vi "dataProcess_spectrZeroOut.vi"(0 "reference":refnum<class "OSA.lvclass">, 1 "spectrum":sgl[](array[numeric]) format="%.2f", 2 "idx start":u32, 3 "idx stop":u32, 4 "length":u32, 5 "error in (no error)":errorcluster) -> (14 "duplicate reference":refnum<class "OSA.lvclass">, 19 "error out":errorcluster)   [LabVIEW 2010, in "OSA.lvclass"]
doc: "This zeros-out a spectrum between the two given indices On return will spectrum be equal to zero at and between the two indices, (idx_start, idx_stop)."
uses:
  OSA.lvclass
  typeDef/xVal_option.ctl
  OSA20X_misc.lvlib
  FTSLib.dll
panel:
  out "spectrum blanked":sgl[](array[numeric]) format="%.2f"
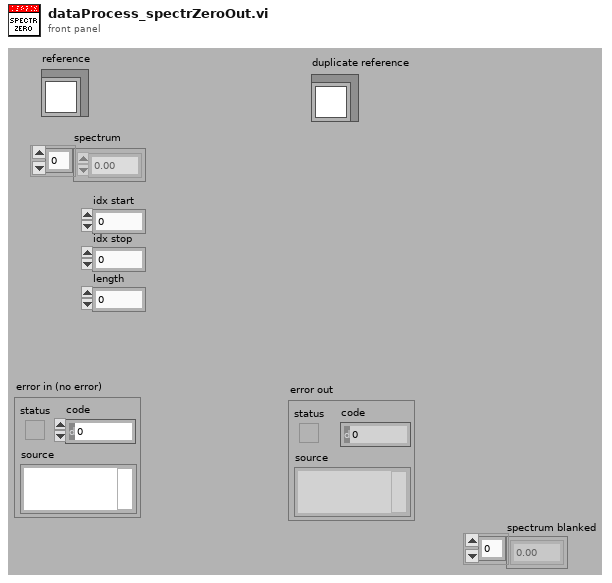
[diagram p1: front panel]
types:
  T1 = typedef "OSA.lvclass/xVal_option.ctl" = enum16{"MIN_MAX", "ARRAY"}
  T2 = cluster{"length":u32, "X min":sgl, "X max":sgl, "X_VAL_OPTIONS":T1}
  T3 = enum16{"get", "init", "set interferogram", "set spectrum", "cleanUp"}
  T4 = typedef "OSA.lvclass/spectrum_properties.ctl" = cluster{"length":u32, "X min":sgl, "X max":sgl, "X_VAL_OPTIONS":T1}
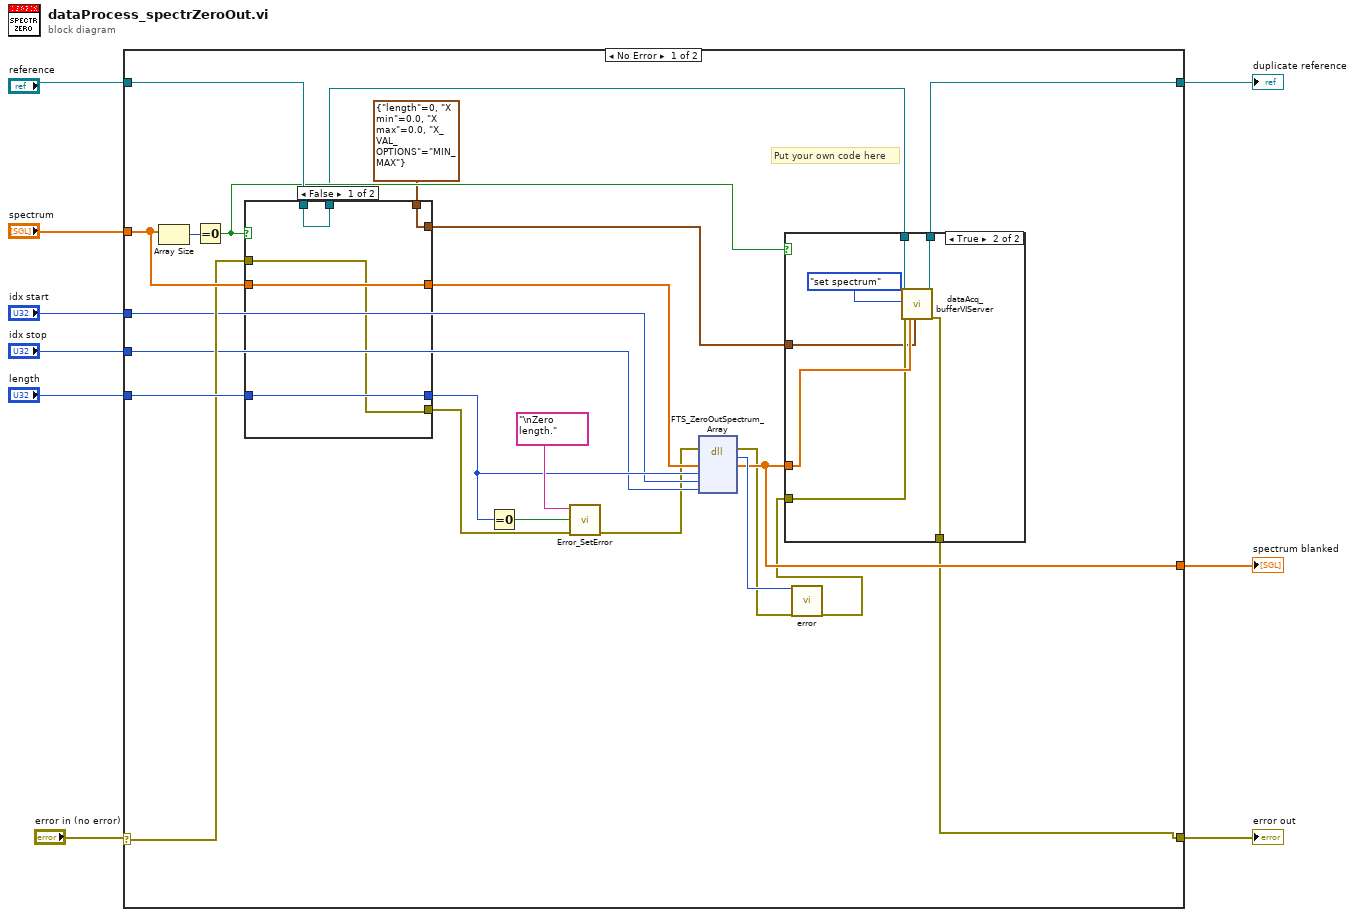
[diagram p0: block diagram]
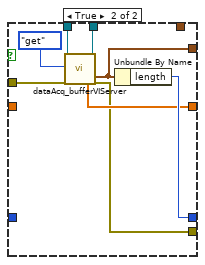
[diagram p3: hidden frame]
diagram:
  n1 = case shown="No Error" "error in (no error)" {
    selector: "error in (no error)" -> [w25 w56]
    tunnel: [w13 w56] -> w9
    tunnel: "reference" -> [w24 w57]
    tunnel: [w17 w57] -> w6
    tunnel: "spectrum" -> [w30 w55]
    tunnel: "idx start" -> [w21 _]
    tunnel: "idx stop" -> [w20 _]
    tunnel: "length" -> [w29 _]
    tunnel: [w16 w55] -> w1
    frame No Error {
      # "Put your own code here"
      n2 = Array Size(array=w30) -> (size(s)=w31:i32)
      n3 = Equal To 0?(x=w31) -> (x = 0?=w19:bool)
      n4 = case shown="False" w19 {
        tunnel: w30 -> [w46 _]
        tunnel: w29 -> [w45 _]
        tunnel: [w46 w50] -> w28
        tunnel: w24 -> [w44 w53]
        tunnel: [w44 w52] -> w18
        tunnel: w25 -> [w43 w48]
        tunnel: [w43 w47] -> w26
        tunnel: [w45 w54] -> w22
        tunnel: [w42 w51] -> w15
        tunnel: T2 {"length"=0, "X min"=0.0, "X max"=0.0, "X_VAL_OPTIONS"=enum."MIN_MAX"} ("spectrum property") -> [w42 _]
        frame False {
        }
        frame True {
          n5 = call "dataAcq_bufferVIServer.vi"("reference"=w53, "action"=T3."get", "error in (no error)"=w48) -> ("spectrum Y"=w50:sgl[], "duplicate reference"=w52:refnum<class "OSA.lvclass">, "spectrum prop"=w51:T4, "error out"=w47:errorcluster)  [unwired: 9 in, 4 out]
          n6 = Unbundle By Name(w51) -> ("length"=w54:u32)
        }
      }
      n7 = Equal To 0?(x=w22) -> (x = 0?=w23:bool)
      n8 = call "Error_SetError.vi"("error in"=w26, "status (true)"=w23, "source(\"\")"="\nZero length." ("source(\"\")")) -> ("error out"=w12:errorcluster)  [unwired: 4 in]
      n9 = dll-call lib="FTSLib.dll" fn="FTS_ZeroOutSpectrum_Array"(error in=w12, "spectrum"=w28, "length"=w22, "startIdx"=w21, "stopIdx"=w20) -> (error out=w11:errorcluster, "return type"=w32:i32, "spectrum"=w16:sgl[])  [unwired: 5 in, 1 out]
      n10 = call "error.vi"("result code"=w32, "error in (no error)"=w11) -> ("error out"=w14:errorcluster)  [unwired: 15 in, 2 out]
      n11 = case shown="True" w19 {
        tunnel: w16 -> [_ w40]
        tunnel: w18 -> [w34 w37]
        tunnel: [w34 w36] -> w17
        tunnel: w15 -> [_ w38]
        tunnel: w14 -> [w33 w39]
        tunnel: [w33 w35] -> w13
        frame False {
        }
        frame True {
          n12 = call "dataAcq_bufferVIServer.vi"("reference"=w37, "action"=T3."set spectrum", "error in (no error)"=w39, "spectrum set Y"=w40, "spectrum prop set"=w38) -> ("duplicate reference"=w36:refnum<class "OSA.lvclass">, "error out"=w35:errorcluster)  [unwired: 7 in, 6 out]
        }
      }
    }
    frame Error {
      # "Error"
    }
  }
  "error out" <- w9
  "duplicate reference" <- w6
  "spectrum blanked" <- w1
